vi "Create CALL msg.vi"(8 "error in":errorcluster, 10 "Call Request":T1, 11 "Request ID":u64) -> (0 "error out":errorcluster, 3 "WAMP Message":string)   [LabVIEW 2020, in "wamplv.lvlib" / "WAMP Client.lvclass"]
uses:
  WAMP Client.lvclass
  TypeDef/WAMP Message Codes.ctl
  API/TypeDefs/WAMP error.ctl
  API/TypeDefs/Combined error.ctl
  API/TypeDefs/RESULT payload.ctl
  TypeDef/CALL Request Data.ctl
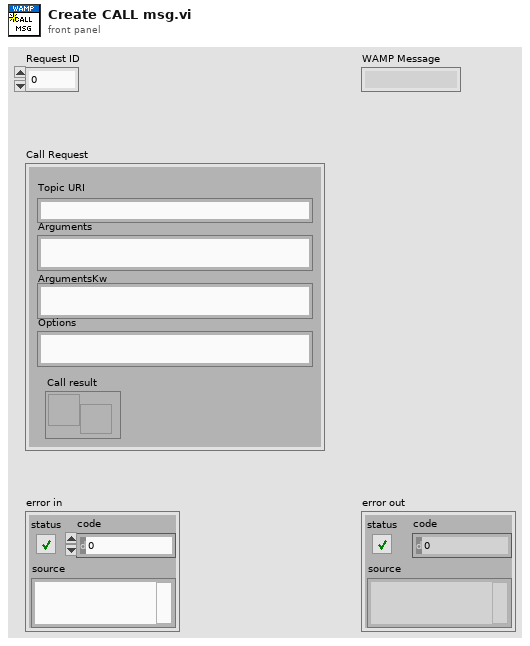
[diagram p1: front panel]
types:
  T1 = typedef "wamplv.lvlib/WAMP Client.lvclass/CALL Request Data.ctl" = cluster{"Topic URI":string, "Arguments":string, "ArgumentsKw":string, "Options":string, "Call result":refnum<notifier>}
  T2 = typedef "wamplv.lvlib/WAMP Client.lvclass/WAMP Message Codes.ctl" = u16
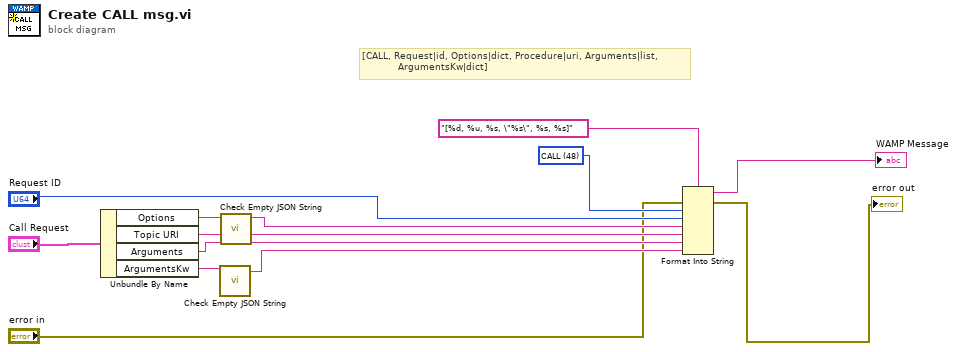
[diagram p0: block diagram]
diagram:
  w6 = T2 48 items=["HELLO"=1, "WELCOME"=2, "ABORT"=3, "GOODBYE"=6, "ERROR"=8, "PUBLISH"=16, "PUBLISHED"=17, "SUBSCRIBE"=32, "SUBSCRIBED"=33, "UNSUBSCRIBE"=34, "UNSUBSCRIBED"=35, "EVENT"=36, "CALL"=48, "RESULT"=59, "REGISTER"=64, "REGISTERED"=65, "UNREGISTER"=66, "UNREGISTERED"=67, "INVOCATION"=68, "YIELD"=70] ("Message Codes")
  # "[CALL, Request|id, Options|dict, Procedure|uri, Arguments|list,\n            ArgumentsKw|dict]"
  n1 = Unbundle By Name("Call Request") -> ("Options"=w11:string, "Topic URI"=w7:string, "Arguments"=w5:string, "ArgumentsKw"=w9:string)
  n2 = call "Check Empty JSON String.vi"("JSON"=w9) -> ("JSON"=w10:string)  [unwired: 10 in]
  n3 = call "Check Empty JSON String.vi"("JSON"=w11) -> ("JSON"=w12:string)  [unwired: 10 in]
  n4 = Format Into String(format string="[%d, %u, %s, \"%s\", %s, %s]" ("element"), error in="error in", w6, "Request ID", w12, w7, w5, w10) -> (resulting string=→"WAMP Message":string, error out=→"error out":errorcluster)  [unwired: 1 in]
